vi "PC-Test1.vi"() -> ()   [LabVIEW 2020]
uses:
  <vilib>/LabVIEW Targets/FPGA/cRIO/shared/nicrio_ModuleControls/nicrio_cRIO-9871_BaudRateEnum.ctl
  <vilib>/LabVIEW Targets/FPGA/cRIO/shared/nicrio_ModuleControls/nicrio_cRIO-9871_DataBitsEnum.ctl
  <vilib>/LabVIEW Targets/FPGA/cRIO/shared/nicrio_ModuleControls/nicrio_cRIO-9871_FlowControlEnum.ctl
  <vilib>/LabVIEW Targets/FPGA/cRIO/shared/nicrio_ModuleControls/nicrio_cRIO-9871_ParityEnum.ctl
  <vilib>/LabVIEW Targets/FPGA/cRIO/shared/nicrio_ModuleControls/nicrio_cRIO-9871_StopBitsEnum.ctl
panel:
  out "Param Errors":u16[](array[numeric]) format="%016b"
  out "Param Settings":u16[](array[numeric]) format="%016b"
  in  "Port# (1-4)":u8=1 min=1 max=4
  in  "Baud Rate 2":T1=enum."9600 bps" caption="Baud"
  in  "Data Bits 2":T2=enum."8"
  in  "Flow Control 2":T3
  in  "Parity 2":T4
  in  "Stop Bits 2":T5
  out "Stop Bits String":string
  out "Parity String":string
  out "Flow Control String":string
  out "Data Bits String":string
  in  "Stop Bits":T5
  in  "Parity":T4
  in  "Flow Control":T3
  in  "Data Bits":T2=enum."8"
  out "Baud Rate String":string
  in  "Baud Rate":T1=enum."9600 bps"
  out "Port on Rx":u16
  out "2nd Nibble HIgh 2 bits  (xxxxNNxx xxxxxxxx)":u8 format="%.0b"
  out "High Nibble Mid 4 bits  (xxNNNNxx xxxxxxxx)":u8 format="%.0b"
  out "Low Byte (xxxxxxxx NNNNNNNN)":u8 format="%.0x"
  out "High Byte (NNNNNNNN xxxxxxxx)":u8 format="%.0x"
  out "High Nibble (NNNNxxxx xxxxxxxx)":u8 format="%.0x"
  in  "U16":u16 format="%.0b"
  out "String":string
  in  "U8#":u8
  # "01AA_AAXX_YYYY_YYYY:\n\nXX - Channel Number, 0-3\nAAAA - UART parameter ID:\n– 0 - Baud rate enumeration. Values are indices\n         in UART baud rate list\n– 1 - Character size. (eg. 5 bits through 8 bits)\n– 2 - Flow control\n– 3 - Parity Check\n– 4 - Number of stop bits. (eg. 1 or 2)\nYYYY_YYYY - Value"
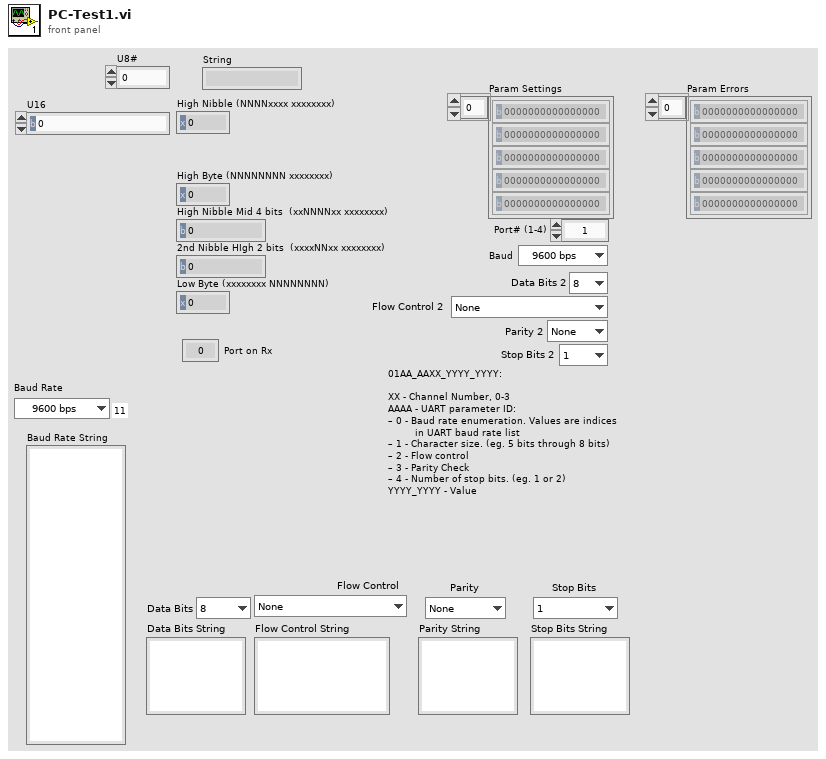
[diagram p1: front panel]
types:
  T1 = typedef "nicrio_cRIO-9871_BaudRateEnum.ctl" = enum16{"75 bps", "110 bps", "134 bps", "150 bps", "300 bps", "600 bps", "1200 bps", "1800 bps", "2400 bps", "4800 bps", "7200 bps", "9600 bps", "14.4 kbps", "19.2 kbps", "28.8 kbps", "38.4 kbps", "57.6 kbps", "115.2 kbps", "230.4 kbps", "460.8 kbps", "921.6 kbps"}
  T2 = typedef "nicrio_cRIO-9871_DataBitsEnum.ctl" = enum8{"5", "6", "7", "8"}
  T3 = typedef "nicrio_cRIO-9871_FlowControlEnum.ctl" = enum8{"None", "Software (XON / XOFF)", "Hardware (RTS / CTS)"}
  T4 = typedef "nicrio_cRIO-9871_ParityEnum.ctl" = enum8{"None", "Odd", "Even", "Mark", "Space"}
  T5 = typedef "nicrio_cRIO-9871_StopBitsEnum.ctl" = enum8{"1", "1.5", "2"}
  T6 = enum16{"TX Byte", "TX Clear", "Echo Request", "Parameter Change"}
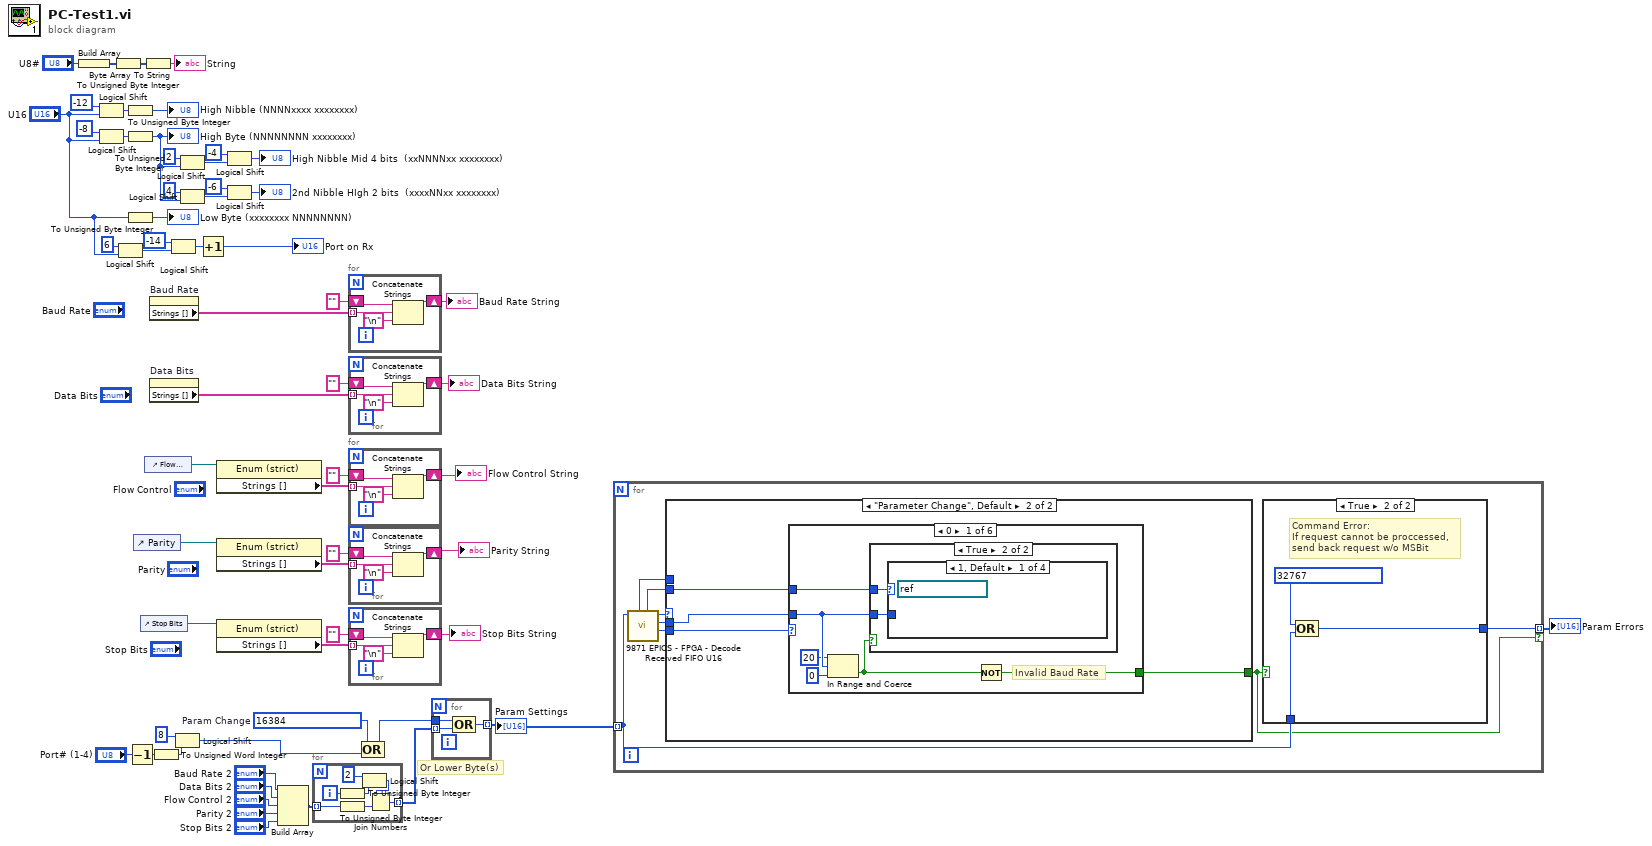
[diagram p0: block diagram]
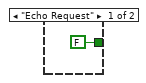
[diagram p3: hidden frame]
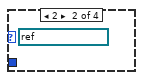
[diagram p5: hidden frame]
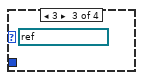
[diagram p6: hidden frame]
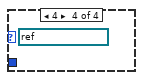
[diagram p7: hidden frame]
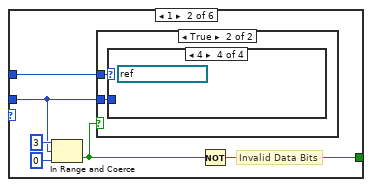
[diagram p8: hidden frame]
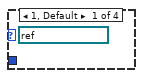
[diagram p10: hidden frame]
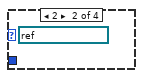
[diagram p11: hidden frame]
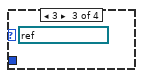
[diagram p12: hidden frame]
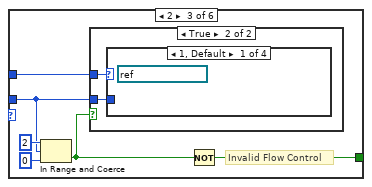
[diagram p13: hidden frame]
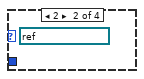
[diagram p15: hidden frame]
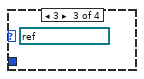
[diagram p16: hidden frame]
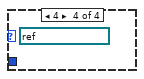
[diagram p17: hidden frame]
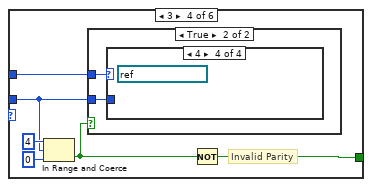
[diagram p18: hidden frame]
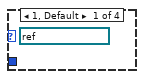
[diagram p20: hidden frame]
diagram:
  w4 = u16 16384  # Param Change
  # "Or Lower Byte(s)"
  n1 = Build Array("U8#") -> (w56:u8[])
  n2 = Logical Shift(y=i16 -12, x="U16") -> (x << y=w54:u16)
  n3 = Logical Shift(y=i16 -8, x="U16") -> (x << y=w53:u16)
  n4 = To Unsigned Byte Integer(number=w56) -> (unsigned 8bit integer=w59:u8[])
  n5 = Logical Shift(y=i16 6, x="U16") -> (x << y=w36:u16)
  n6 = To Unsigned Byte Integer(number=w54) -> (unsigned 8bit integer=→"High Nibble (NNNNxxxx xxxxxxxx)":u8)
  n7 = To Unsigned Byte Integer(number=w53) -> (unsigned 8bit integer=w41:u8)
  "High Byte (NNNNNNNN xxxxxxxx)" <- w41
  n8 = To Unsigned Byte Integer(number="U16") -> (unsigned 8bit integer=→"Low Byte (xxxxxxxx NNNNNNNN)":u8)
  n9 = Decrement(x="Port# (1-4)") -> (x-1=w13:u8)
  n10 = control-ref of="Parity"() -> (w21:refnum<vi>)
  n11 = control-ref of="Stop Bits"() -> (w20:refnum<vi>)
  n12 = Byte Array To String(unsigned byte array=w59) -> (string=→"String":string)
  n13 = control-ref of="Flow Control"() -> (w22:refnum<vi>)
  n14 = property on="Baud Rate" class="Enum (strict)"() -> ("Strings []"=w34:string[])  [unwired: 2 in, 2 out]
  n15 = property on="Data Bits" class="Enum (strict)"() -> ("Strings []"=w30:string[])  [unwired: 2 in, 2 out]
  n16 = To Unsigned Word Integer(number=w13) -> (unsigned 16bit integer=w15:u16)
  n17 = Logical Shift(y=i16 -14, x=w36) -> (x << y=w35:u16)
  n18 = Logical Shift(y=i16 8, x=w15) -> (x << y=w11:u16)
  n19 = Logical Shift(y=i16 2, x=w41) -> (x << y=w47:u8)
  n20 = Logical Shift(y=i16 4, x=w41) -> (x << y=w44:u8)
  n21 = Increment(x=w35) -> (x+1=→"Port on Rx":u16)
  n22 = property on="Property Node" class="Enum (strict)"(reference=w22) -> ("Strings []"=w27:string[])  [unwired: 1 in, 2 out]
  n23 = property on="Property Node" class="Enum (strict)"(reference=w21) -> ("Strings []"=w26:string[])  [unwired: 1 in, 2 out]
  n24 = property on="Property Node" class="Enum (strict)"(reference=w20) -> ("Strings []"=w23:string[])  [unwired: 1 in, 2 out]
  n25 = Logical Shift(y=i16 -4, x=w47) -> (x << y=→"High Nibble Mid 4 bits  (xxNNNNxx xxxxxxxx)":u8)
  n26 = Logical Shift(y=i16 -6, x=w44) -> (x << y=→"2nd Nibble HIgh 2 bits  (xxxxNNxx xxxxxxxx)":u8)
  n27 = Build Array("Baud Rate 2", "Data Bits 2", "Flow Control 2", "Parity 2", "Stop Bits 2") -> (w10:u16[])
  n28 = for {
    tunnel: w10 -> [w66] mode=indexing
    tunnel: [w63] -> w3 mode=indexing
    i -> [w64]
    n29 = To Unsigned Byte Integer(number=w64) -> (unsigned 8bit integer=w60:u8)
    n30 = To Unsigned Byte Integer(number=w66) -> (unsigned 8bit integer=w65:u8)
    n31 = Logical Shift(y=i16 2, x=w60) -> (x << y=w61:u8)
    n32 = Join Numbers(hi=w61, lo=w65) -> ((hi.lo)=w63:u16)
  }
  n33 = for {
    tunnel: w34 -> [w70] mode=indexing
    shift-right: [w68] -> w32
    shift-left: "" -> [w67]
    n34 = Concatenate Strings(w67, w70, "\n" ("string")) -> (w68:string)
  }
  "Baud Rate String" <- w32
  n35 = for {
    tunnel: w30 -> [w74] mode=indexing
    shift-right: [w72] -> w29
    shift-left: "" -> [w71]
    n36 = Concatenate Strings(w71, w74, "\n" ("string")) -> (w72:string)
  }
  "Data Bits String" <- w29
  n37 = for {
    tunnel: w27 -> [w78] mode=indexing
    shift-right: [w76] -> w19
    shift-left: "" -> [w75]
    n38 = Concatenate Strings(w75, w78, "\n" ("string")) -> (w76:string)
  }
  "Flow Control String" <- w19
  n39 = for {
    tunnel: w26 -> [w82] mode=indexing
    shift-right: [w80] -> w18
    shift-left: "" -> [w79]
    n40 = Concatenate Strings(w79, w82, "\n" ("string")) -> (w80:string)
  }
  "Parity String" <- w18
  n41 = for {
    tunnel: w23 -> [w86] mode=indexing
    shift-right: [w84] -> w17
    shift-left: "" -> [w83]
    n42 = Concatenate Strings(w83, w86, "\n" ("string")) -> (w84:string)
  }
  "Stop Bits String" <- w17
  n43 = Compound Arithmetic op=OR(w4, w11) -> (w16:u16)
  n44 = for {
    tunnel: w3 -> [w87] mode=indexing
    tunnel: [w89] -> w2 mode=indexing
    tunnel: w16 -> [w88]
    n45 = Compound Arithmetic op=OR(w88, w87) -> (w89:u16)
  }
  "Param Settings" <- w2
  n46 = for {
    tunnel: w2 -> [w97] mode=indexing
    tunnel: [w91] -> w1 mode=indexing if=w90
    n47 = call "9871 EPICS - FPGA - Decode Received FIFO U16.vi"("U16"=w97) -> ("Parameter High Nibble Mid 4 bits  (xxNNNNxx xxxxxxxx)"=w92:u8, "Low Byte (xxxxxxxx NNNNNNNN)"=w95:u8, "Request Type"=w96:T6, "Port# (1-4)"=w94:u8, "Port Bits Only in U16"=w93:u16)  [unwired: 6 in]
    n48 = case shown="\"Parameter Change\", Default" w96 {
      tunnel: w95 -> [_ w105]
      tunnel: w94 -> [_ w103]
      tunnel: w93 -> [_ _]
      tunnel: w92 -> [_ w104]
      tunnel: [FALSE w102] -> w90
      frame "Echo Request" {
      }
      frame "Parameter Change", Default {
        n49 = case shown="0" w104 {
          tunnel: w105 -> [w110 w116 w124 w131 w140 _]
          tunnel: [w106 w115 w123 w132 w139 w146] -> w102
          tunnel: w103 -> [w111 w119 w127 w135 w143 _]
          frame 0 {
            # "Invalid Baud Rate"
            n50 = In Range and Coerce(upper limit=u8 20, x=w110, lower limit=u8 0) -> (In Range?=w107:bool)  [unwired: 1 out]
            n51 = case shown="True" w107 {
              tunnel: w111 -> [_ w113]
              tunnel: w110 -> [_ w112]
              frame False {
              }
              frame True {
                n52 = case shown="1, Default" w113 {
                  tunnel: w112 -> [_ _ _ _]
                  frame 1, Default {
                    (unwired) refnum<k21> "9871A\\Port1" ("cRIO I/O Device")
                  }
                  frame 2 {
                    (unwired) refnum<k21> "9871A\\Port2" ("cRIO I/O Device")
                  }
                  frame 3 {
                    (unwired) refnum<k21> "9871A\\Port3" ("cRIO I/O Device")
                  }
                  frame 4 {
                    (unwired) refnum<k21> "9871A\\Port4" ("cRIO I/O Device")
                  }
                }
              }
            }
            n53 = Not(x=w107) -> (.not. x?=w106:bool)
          }
          frame 1 {
            # "Invalid Data Bits"
            n54 = In Range and Coerce(upper limit=u8 3, x=w116, lower limit=u8 0) -> (In Range?=w114:bool)  [unwired: 1 out]
            n55 = case shown="True" w114 {
              tunnel: w119 -> [_ w121]
              tunnel: w116 -> [_ w120]
              frame False {
              }
              frame True {
                n56 = case shown="4" w121 {
                  tunnel: w120 -> [_ _ _ _]
                  frame 1, Default {
                    (unwired) refnum<k21> "9871A\\Port1" ("cRIO I/O Device")
                  }
                  frame 2 {
                    (unwired) refnum<k21> "9871A\\Port2" ("cRIO I/O Device")
                  }
                  frame 3 {
                    (unwired) refnum<k21> "9871A\\Port3" ("cRIO I/O Device")
                  }
                  frame 4 {
                    (unwired) refnum<k21> "9871A\\Port4" ("cRIO I/O Device")
                  }
                }
              }
            }
            n57 = Not(x=w114) -> (.not. x?=w115:bool)
          }
          frame 2 {
            # "Invalid Flow Control"
            n58 = In Range and Coerce(upper limit=u8 2, x=w124, lower limit=u8 0) -> (In Range?=w122:bool)  [unwired: 1 out]
            n59 = case shown="True" w122 {
              tunnel: w127 -> [_ w129]
              tunnel: w124 -> [_ w128]
              frame False {
              }
              frame True {
                n60 = case shown="1, Default" w129 {
                  tunnel: w128 -> [_ _ _ _]
                  frame 1, Default {
                    (unwired) refnum<k21> "9871A\\Port1" ("cRIO I/O Device")
                  }
                  frame 2 {
                    (unwired) refnum<k21> "9871A\\Port2" ("cRIO I/O Device")
                  }
                  frame 3 {
                    (unwired) refnum<k21> "9871A\\Port3" ("cRIO I/O Device")
                  }
                  frame 4 {
                    (unwired) refnum<k21> "9871A\\Port4" ("cRIO I/O Device")
                  }
                }
              }
            }
            n61 = Not(x=w122) -> (.not. x?=w123:bool)
          }
          frame 3 {
            # "Invalid Parity"
            n62 = In Range and Coerce(upper limit=u8 4, x=w131, lower limit=u8 0) -> (In Range?=w130:bool)  [unwired: 1 out]
            n63 = case shown="True" w130 {
              tunnel: w135 -> [_ w137]
              tunnel: w131 -> [_ w136]
              frame False {
              }
              frame True {
                n64 = case shown="4" w137 {
                  tunnel: w136 -> [_ _ _ _]
                  frame 1, Default {
                    (unwired) refnum<k21> "9871A\\Port1" ("cRIO I/O Device")
                  }
                  frame 2 {
                    (unwired) refnum<k21> "9871A\\Port2" ("cRIO I/O Device")
                  }
                  frame 3 {
                    (unwired) refnum<k21> "9871A\\Port3" ("cRIO I/O Device")
                  }
                  frame 4 {
                    (unwired) refnum<k21> "9871A\\Port4" ("cRIO I/O Device")
                  }
                }
              }
            }
            n65 = Not(x=w130) -> (.not. x?=w132:bool)
          }
          frame 4 {
            # "Invalid Stop Bits"
            n66 = In Range and Coerce(upper limit=u8 2, x=w140, lower limit=u8 0) -> (In Range?=w138:bool)  [unwired: 1 out]
            n67 = case shown="True" w138 {
              tunnel: w143 -> [_ w145]
              tunnel: w140 -> [_ w144]
              frame False {
              }
              frame True {
                n68 = case shown="4" w145 {
                  tunnel: w144 -> [_ _ _ _]
                  frame 1, Default {
                    (unwired) refnum<k21> "9871A\\Port1" ("cRIO I/O Device")
                  }
                  frame 2 {
                    (unwired) refnum<k21> "9871A\\Port2" ("cRIO I/O Device")
                  }
                  frame 3 {
                    (unwired) refnum<k21> "9871A\\Port3" ("cRIO I/O Device")
                  }
                  frame 4 {
                    (unwired) refnum<k21> "9871A\\Port4" ("cRIO I/O Device")
                  }
                }
              }
            }
            n69 = Not(x=w138) -> (.not. x?=w139:bool)
          }
          frame 5.. {
            w146 = TRUE  # Invalid UART Parameter ID
          }
        }
      }
    }
    n70 = case shown="True" w90 {
      tunnel: w97 -> [_ w100]
      tunnel: [_ w98] -> w91
      frame False {
      }
      frame True {
        # "Command Error:\nIf request cannot be proccessed,\nsend back request w/o MSBit"
        n71 = Compound Arithmetic op=OR(u16 32767, w100) -> (w98:u16)
      }
    }
  }
  "Param Errors" <- w1
